vi "set_triggerable.vi"(8 "error in (no error)":errorcluster, 10 "triggerable?":bool, 11 "GenericDAQ in":refnum<class "GenericDAQ.lvclass">) -> (0 "error out":errorcluster, 3 "GenericDAQ out":refnum<class "GenericDAQ.lvclass">)   [LabVIEW 2010, in "GenericDAQ.lvclass"]
uses:
  GenericDAQ.lvclass
  GenericDAQ.lvclass/GenericDAQ.ctl
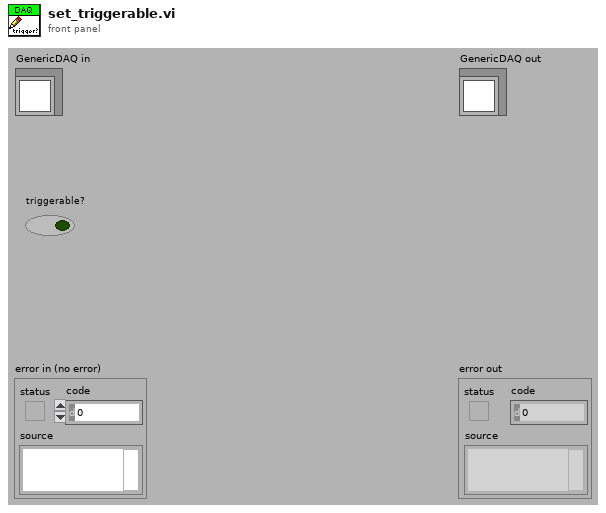
[diagram p1: front panel]
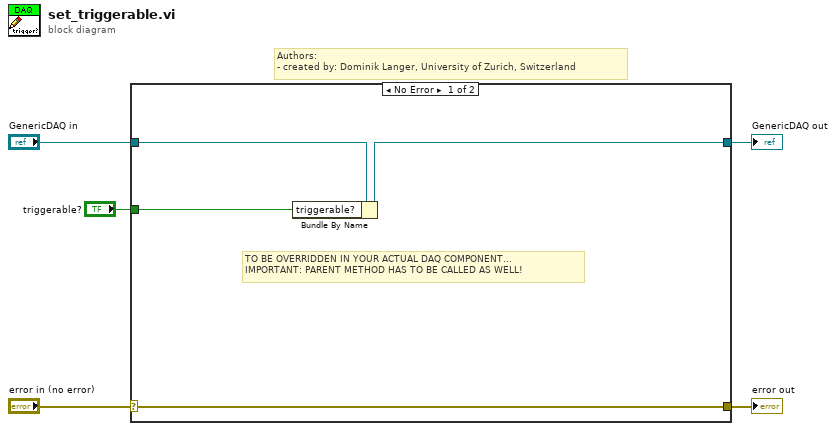
[diagram p0: block diagram]
diagram:
  # "Authors: \n- created by: Dominik Langer, University of Zurich, Switzerland"
  n1 = case shown="No Error" "error in (no error)" {
    selector: "error in (no error)" -> [w9 w11]
    tunnel: [w9 w11] -> w4
    tunnel: [w7 w10] -> w2
    tunnel: "GenericDAQ in" -> [w8 w10]
    tunnel: "triggerable?" -> [w6 _]
    frame No Error {
      # "TO BE OVERRIDDEN IN YOUR ACTUAL DAQ COMPONENT...\nIMPORTANT: PARENT METHOD HAS TO BE CALLED AS WELL!"
      n2 = Bundle By Name(cluster=w8, "triggerable?"=w6) -> (w7:refnum<class "GenericDAQ.lvclass">)
    }
    frame Error {
    }
  }
  "error out" <- w4
  "GenericDAQ out" <- w2
